vi "Log Event.vi"(8 "error in (no error)":cluster{"状态":bool, "代码":i32, "源":string} caption="错误输入（无错误）", 10 "事件文本":string, 11 "多任务通讯输入":refnum<class "多任务通讯.lvclass">) -> (0 "error out":cluster{"状态":bool, "代码":i32, "源":string} caption="错误输出")   [LabVIEW 2013, in "多任务通讯.lvlib" / "多任务通讯.lvclass"]
doc: "向当前事件记录添加文本。"
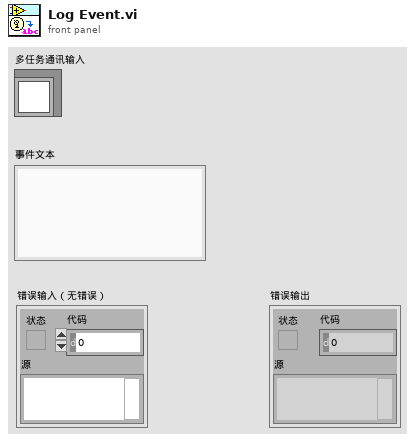
[diagram p1: front panel]
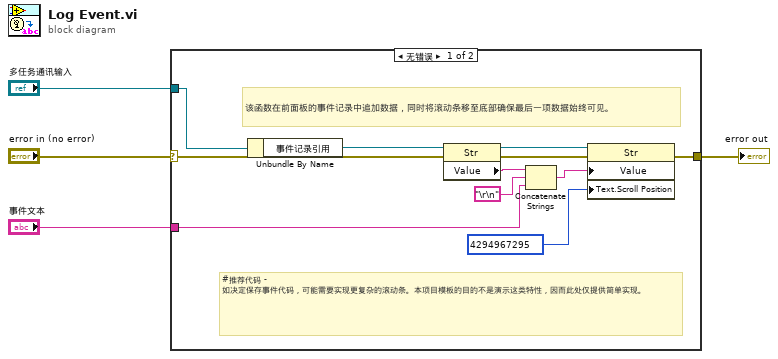
[diagram p0: block diagram]
diagram:
  n1 = case shown="无错误" "error in (no error)" {
    selector: "error in (no error)" -> [w7 w16]
    tunnel: [w8 w16] -> w3
    tunnel: "多任务通讯输入" -> [w15 _]
    tunnel: "事件文本" -> [w12 _]
    frame No Error {
      # "#推荐代码 - 如决定保存事件代码，可能需要实现更复杂的滚动条。本项目模板的目的不是演示这类特性，因而此处仅提供简单实现。"
      # "该函数在前面板的事件记录中追加数据，同时将滚动条移至底部确保最后一项数据始终可见。"
      n2 = Unbundle By Name(w15) -> ("事件记录引用"=w14:refnum<vi>)
      n3 = property class="Str"(reference=w14, error in=w7) -> (reference out=w10:refnum<vi>, error out=w9:errorcluster, "Value"=w13:string)
      n4 = Concatenate Strings(w13, "\r\n", w12) -> (w6:string)
      n5 = property class="Str"(reference=w10, error in=w9, "Value"=w6, "Text.Scroll Position"=u32 4294967295) -> (error out=w8:errorcluster)  [unwired: 1 out]
    }
    frame Error {
    }
  }
  "error out" <- w3
